vi "classify type.vi"(11 "data type":T1) -> (2 "array?":bool, 3 "numeric?":bool)   [LabVIEW 2013, in "tag bus.lvlib" / "tag descriptor.lvclass"]
uses:
  tag descriptor.lvclass
  Data Type.ctl
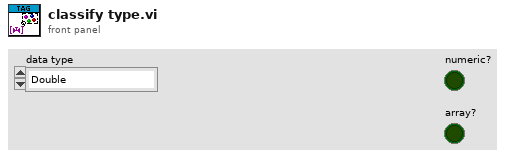
[diagram p1: front panel]
types:
  T1 = typedef "tag bus.lvlib/tag descriptor.lvclass/Data Type.ctl" = enum16{"Double", "Single", "I64", "I32", "I16", "I8", "U64", "U32", "U16", "U8", "Boolean", "String", "Array of Double", "Array of Single", "Array of I64", "Array of I32", "Array of I16", "Array of I8", "Array of U64", "Array of U32", "Array of U16", "Array of U8", "Array of Boolean", "Array of String"}
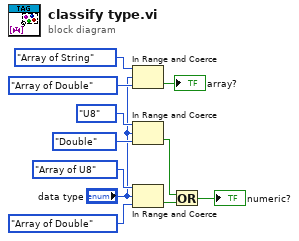
[diagram p0: block diagram]
diagram:
  n1 = In Range and Coerce(upper limit=Data_Type."Array of String", x="data type", lower limit=Data_Type."Array of Double") -> (In Range?=→"array?":bool)  [unwired: 1 out]
  n2 = In Range and Coerce(upper limit=Data_Type."U8", x="data type", lower limit=Data_Type."Double") -> (In Range?=w6:bool)  [unwired: 1 out]
  n3 = In Range and Coerce(upper limit=Data_Type."Array of U8", x="data type", lower limit=Data_Type."Array of Double") -> (In Range?=w7:bool)  [unwired: 1 out]
  n4 = Or(x=w6, y=w7) -> (x .or. y?=→"numeric?":bool)
